vi "U642Bin.vi"(11 "数值":u64) -> (2 "输出簇":T1)   [LabVIEW 2019]
panel:
  out "布尔数组":bool[](array[boolean])
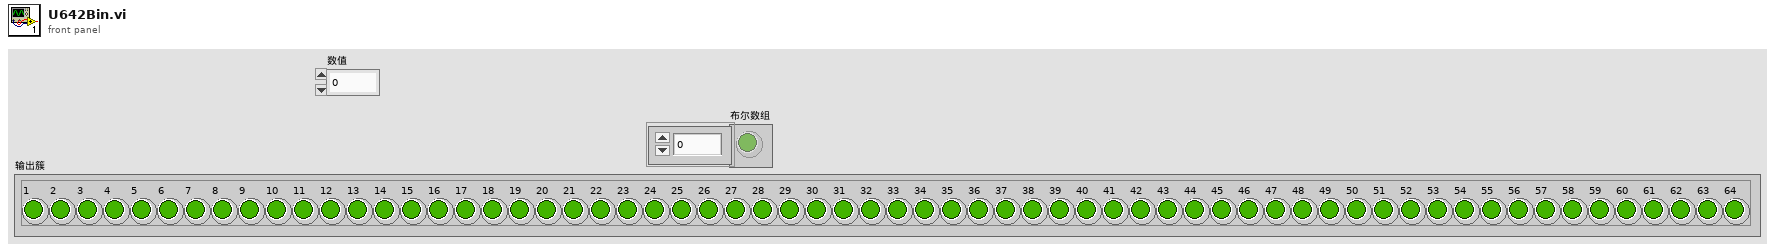
[diagram p1: front panel]
types:
  T1 = cluster{"1":bool, "2":bool, "3":bool, "4":bool, "5":bool, "6":bool, "7":bool, "8":bool, "9":bool, "10":bool, "11":bool, "12":bool, "13":bool, "14":bool, "15":bool, "16":bool, "17":bool, "18":bool, "19":bool, "20":bool, "21":bool, "22":bool, "23":bool, "24":bool, "25":bool, "26":bool, "27":bool, "28":bool, "29":bool, "30":bool, "31":bool, "32":bool, "33":bool, "34":bool, "35":bool, "36":bool, "37":bool, "38":bool, "39":bool, "40":bool, "41":bool, "42":bool, "43":bool, "44":bool, "45":bool, "46":bool, "47":bool, "48":bool, "49":bool, "50":bool, "51":bool, "52":bool, "53":bool, "54":bool, "55":bool, "56":bool, "57":bool, "58":bool, "59":bool, "60":bool, "61":bool, "62":bool, "63":bool, "64":bool}
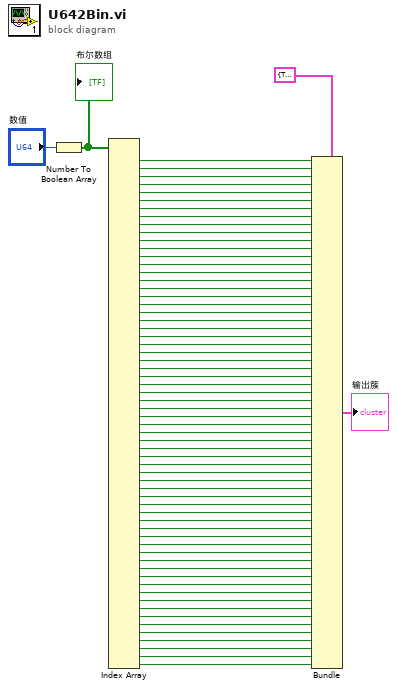
[diagram p0: block diagram]
diagram:
  n1 = Number To Boolean Array(number="数值") -> (Boolean array=w67:bool[])
  "布尔数组" <- w67
  n2 = Index Array(array=w67) -> (element #1=w66:bool, element #2=w65:bool, element #3=w64:bool, element #4=w63:bool, element #5=w62:bool, element #6=w61:bool, element #7=w60:bool, element #8=w59:bool, element #9=w57:bool, element #10=w56:bool, element #11=w55:bool, element #12=w53:bool, element #13=w52:bool, element #14=w51:bool, element #15=w50:bool, element #16=w49:bool, element #17=w48:bool, element #18=w47:bool, element #19=w46:bool, element #20=w45:bool, element #21=w43:bool, element #22=w42:bool, element #23=w41:bool, element #24=w40:bool, element #25=w39:bool, element #26=w38:bool, element #27=w37:bool, element #28=w36:bool, element #29=w35:bool, element #30=w34:bool, element #31=w33:bool, element #32=w32:bool, element #33=w31:bool, element #34=w30:bool, element #35=w29:bool, element #36=w28:bool, element #37=w27:bool, element #38=w26:bool, element #39=w25:bool, element #40=w24:bool, element #41=w23:bool, element #42=w22:bool, element #43=w21:bool, element #44=w20:bool, element #45=w19:bool, element #46=w18:bool, element #47=w17:bool, element #48=w16:bool, element #49=w15:bool, element #50=w14:bool, element #51=w13:bool, element #52=w12:bool, element #53=w11:bool, element #54=w10:bool, element #55=w9:bool, element #56=w8:bool, element #57=w7:bool, element #58=w6:bool, element #59=w5:bool, element #60=w4:bool, element #61=w3:bool, element #62=w2:bool, element #63=w1:bool, element #64=w44:bool)  [unwired: 64 in]
  n3 = Bundle(cluster=T1 {"1"=TRUE, "2"=TRUE, "3"=TRUE, "4"=TRUE, "5"=TRUE, "6"=TRUE, "7"=TRUE, "8"=TRUE, "9"=TRUE, "10"=TRUE, "11"=TRUE, "12"=TRUE, "13"=TRUE, "14"=TRUE, "15"=TRUE, "16"=TRUE, "17"=TRUE, "18"=TRUE, "19"=TRUE, "20"=TRUE, "21"=TRUE, "22"=TRUE, "23"=TRUE, "24"=TRUE, "25"=TRUE, "26"=TRUE, "27"=TRUE, "28"=TRUE, "29"=TRUE, "30"=TRUE, "31"=TRUE, "32"=TRUE, "33"=TRUE, "34"=TRUE, "35"=TRUE, "36"=TRUE, "37"=TRUE, "38"=TRUE, "39"=TRUE, "40"=TRUE, "41"=TRUE, "42"=TRUE, "43"=TRUE, "44"=TRUE, "45"=TRUE, "46"=TRUE, "47"=TRUE, "48"=TRUE, "49"=TRUE, "50"=TRUE, "51"=TRUE, "52"=TRUE, "53"=TRUE, "54"=TRUE, "55"=TRUE, "56"=TRUE, "57"=TRUE, "58"=TRUE, "59"=TRUE, "60"=TRUE, "61"=TRUE, "62"=TRUE, "63"=TRUE, "64"=TRUE}, "1"=w66, "2"=w65, "3"=w64, "4"=w63, "5"=w62, "6"=w61, "7"=w60, "8"=w59, "9"=w57, "10"=w56, "11"=w55, "12"=w53, "13"=w52, "14"=w51, "15"=w50, "16"=w49, "17"=w48, "18"=w47, "19"=w46, "20"=w45, "21"=w43, "22"=w42, "23"=w41, "24"=w40, "25"=w39, "26"=w38, "27"=w37, "28"=w36, "29"=w35, "30"=w34, "31"=w33, "32"=w32, "33"=w31, "34"=w30, "35"=w29, "36"=w28, "37"=w27, "38"=w26, "39"=w25, "40"=w24, "41"=w23, "42"=w22, "43"=w21, "44"=w20, "45"=w19, "46"=w18, "47"=w17, "48"=w16, "49"=w15, "50"=w14, "51"=w13, "52"=w12, "53"=w11, "54"=w10, "55"=w9, "56"=w8, "57"=w7, "58"=w6, "59"=w5, "60"=w4, "61"=w3, "62"=w2, "63"=w1, "64"=w44) -> (→"输出簇":T1)
